vi "OA Get Mode Acq Params.vi"(10 "pcListOfParams":string, 11 "pcModeName":string) -> (2 "pcListOfParams out":string, 3 "function return":u32)   [LabVIEW 2018, in "AndorSDK.lvlib"]
doc: "EXPNETTYPE unsigned int WINAPI OA_GetModeAcqParams(const char * const pcModeName, char * const pcListOfParams);"
uses:
  AndorSDK.lvlib
  ATMCD32D.dll
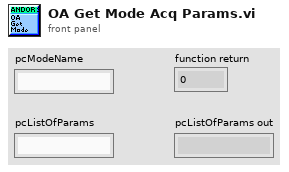
[diagram p1: front panel]
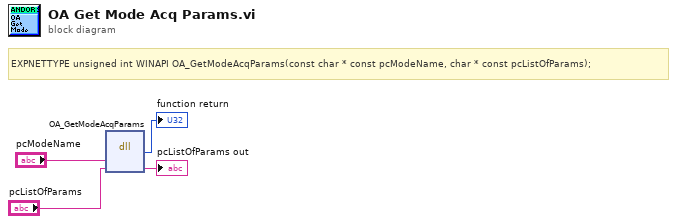
[diagram p0: block diagram]
diagram:
  # "EXPNETTYPE unsigned int WINAPI OA_GetModeAcqParams(const char * const pcModeName, char * const pcListOfParams);"
  n1 = dll-call lib="PTH2babs E\nPersönliches02 - Arbeit03-HiwijobsLabviewCodelibANDOR\tAndor SDK\nATMCD32D.*" fn="OA_GetModeAcqParams"("pcModeName"="pcModeName", "pcListOfParams"="pcListOfParams") -> (→"function return":u32, "pcListOfParams"=→"pcListOfParams out":string)  [unwired: 4 in, 2 out]
